vi "Load DLL into memory.vi"() -> (0 "error out":errorcluster, 3 "path out":path=path "C:/Snap-On_M4/trunk/Software/Code Modules/DLL/ScopeTestDll.dll")   [LabVIEW 2013]
panel:
  out "return type":i32
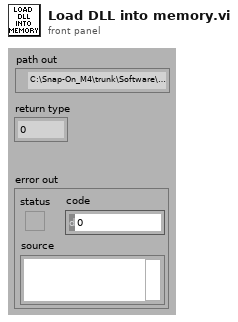
[diagram p1: front panel]
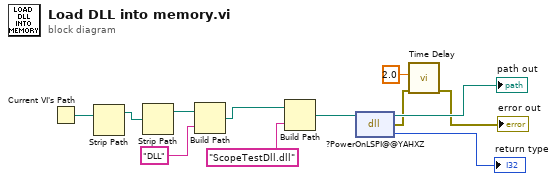
[diagram p0: block diagram]
diagram:
  n1 = Current VI's Path() -> (path=w12:path)
  n2 = Strip Path(path=w12) -> (stripped path=w11:path)  [unwired: 1 out]
  n3 = Strip Path(path=w11) -> (stripped path=w10:path)  [unwired: 1 out]
  n4 = Build Path(base path=w10, name or relative path="DLL") -> (appended path=w6:path)
  n5 = Build Path(base path=w6, name or relative path="ScopeTestDll.dll") -> (appended path=w8:path)
  n6 = dll-call lib="C:/Snap-On_M4/trunk/Software/Code Modules/DLL/ScopeTestDll.dll" fn="?PowerOnLSPI@@YAHXZ"(path in=w8) -> (path out=→"path out":path, error out=w2:errorcluster, "return type"=→"return type":i32)  [unwired: 2 in]
  n7 = call "Time Delay"("error in (no error)"=w2, "Delay Time (s)"=2.0) -> ("error out"=→"error out":errorcluster)  [unwired: 9 in]
